vi "pco.camera_Simple_Example.vi"() -> ()   [LabVIEW 2019]
uses:
  pco.camera/Camera.lvclass
  <vilib>/picture/picture.llb/Draw 8-Bit Pixmap.vi
  <vilib>/picture/picture.llb/Draw True-Color Pixmap.vi
panel:
  out "colormap(U8)":u32[](array[numeric])
  out "Image(U16)":u16[][](graph)
  in  "Zoom [%]":i32(c297)=26
  out "Image":picture
  out "rawImage":u16[][](array[numeric])
  in  "data_format":T1(ring)=enum."Mono16"
  in  "Image Index":u32 max=9
  out "Recorded Images":u32
  in  "Quit":bool
  in  "roiY1":u64=2 min=2 max=2160 step=1
  in  "roiX1":u64=2 min=2 max=2560 step=1
  in  "roiY0":u64=1 min=1 max=2159 step=1
  in  "roiX0":u64=1 min=1 max=2559 step=1
  out "Image Height":u16
  out "Image Width":u16
  in  "dwImgCount":u32=10 caption="Required Number of Images" max=4023
  out "Error":errorcluster {"code" format="%x"}
  # "This example shows a simple recording of an image sequence and the image access afterwards.\nIt is a good starting point for writing own applications.\nBut it will not be fail save, i.e. doesnt react on errors, just handles them forward to the end\n\nUsage:\nSelect your required image count before you start the program.\nOnce started, the camera class will be initialized and images will be recorded automatically.\nWhen acquisition has finished you can address the images and set a certain roi \nTo finish the program click on quit application, this will force fan exit of the camera class"
  # "pco.labview"
  # "Camera Setup"
  # "Recording Control"
  # "Parameters for image readout"
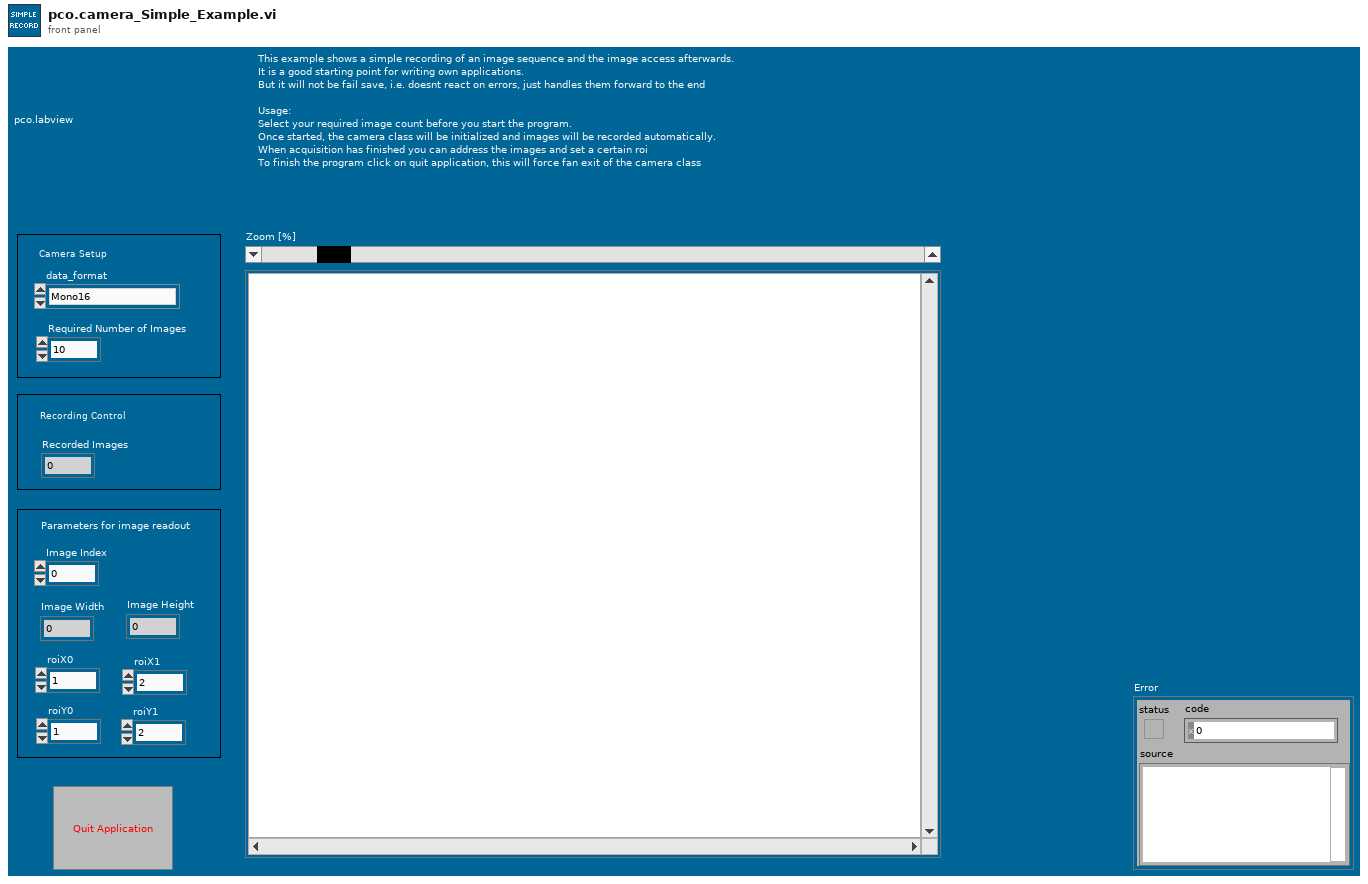
[diagram p1: front panel]
types:
  T1 = enum16{"Undefined", "Mono8", "Mono16", "BGRA8", "RGBA8", "BGRA16", "RGBA16", "CompressedMono8"}
  T2 = enum8{"Enabled", "Disabled", "Disabled and Grayed Out"}
  T3 = enum16{"sequence", "sequence non blocking", "ring buffer", "fifo", "sequence_dpcore", "sequence_non_blocking_dpcore", "ring_buffer_dpcore", "fifo_dpcore", "tif", "multitif", "pcoraw", "b16", "dicom", "multidicom"}
  T4 = typedef "Camera.lvclass/binning.ctl" = cluster{"vert":u16, "horz":u16}
  T5 = cluster{"exposure_time_s":dbl, "delay_time_s":dbl, "roi":cluster{"x0":u64, "y0":u64, "x1":u64, "y1":u64}, "timestamp_mode":u16, "pixelrate":u32, "trigger_mode":u16, "acquire_mode":u16, "metadata_mode":u16, "noisefilter_mode":u16, "binning":T4}
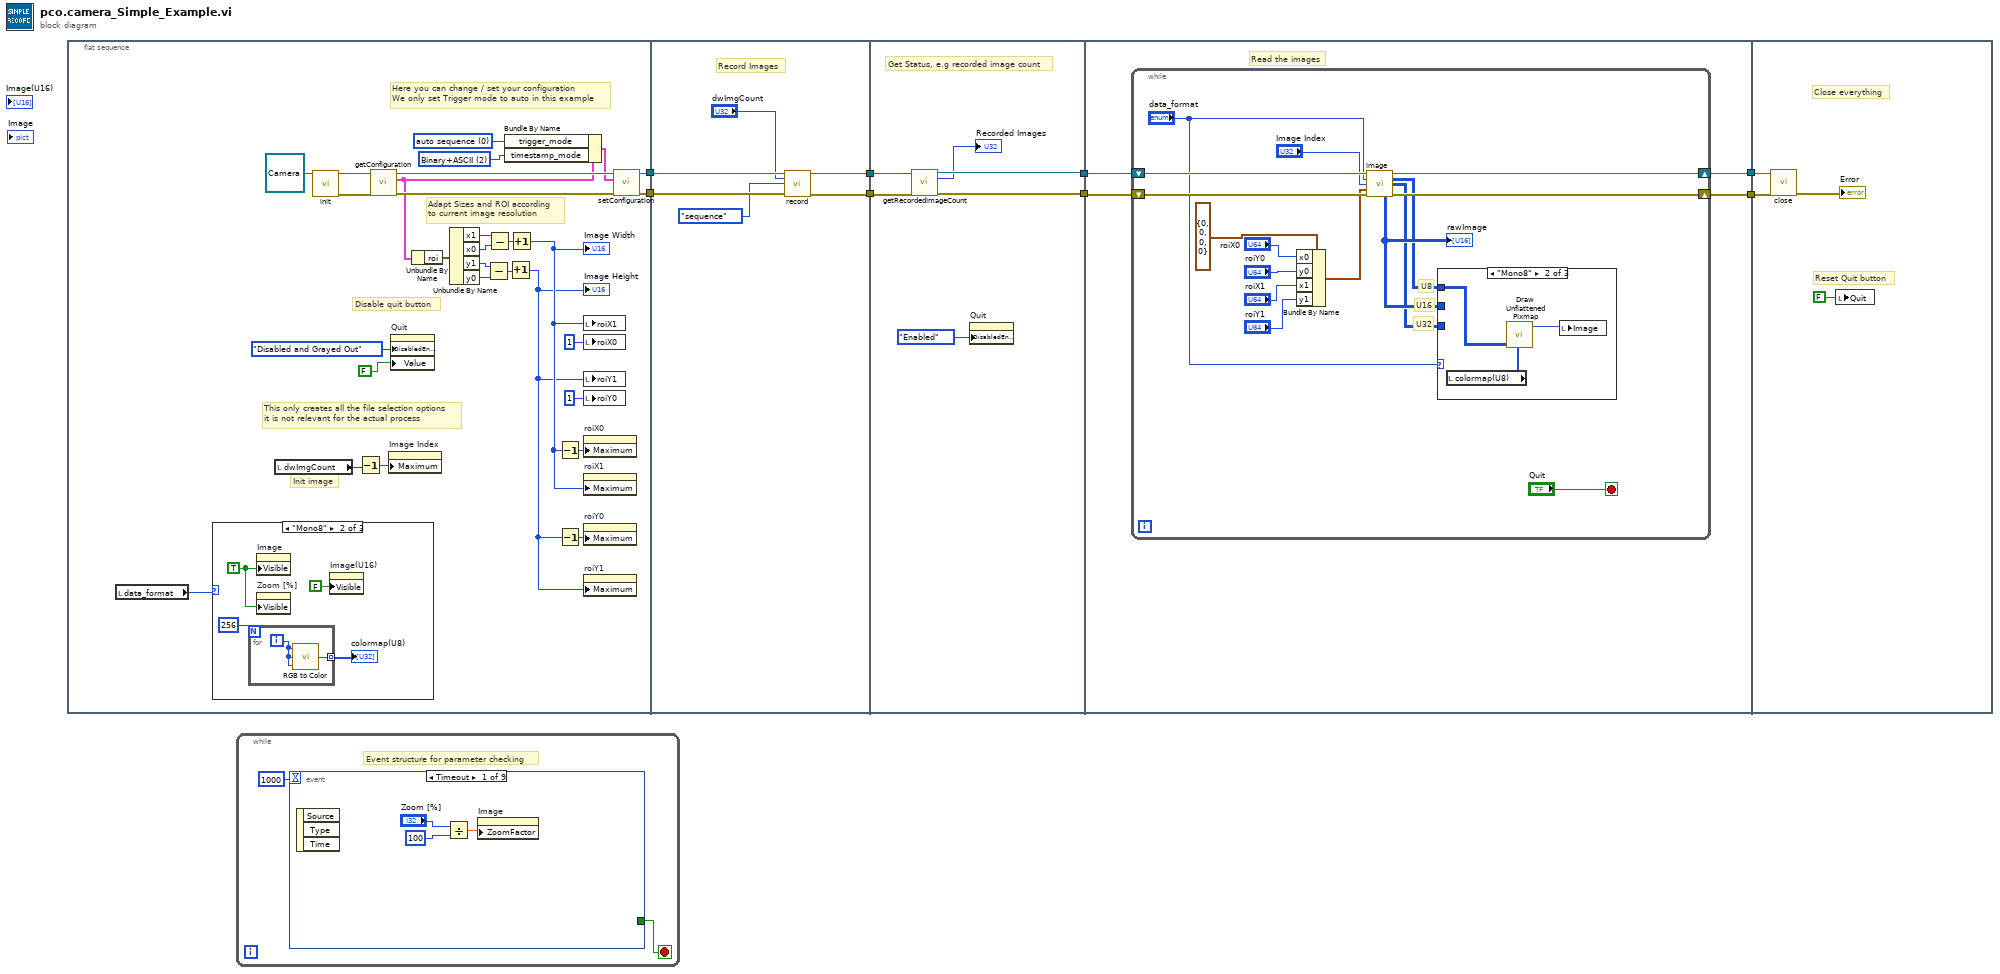
[diagram p0: block diagram]
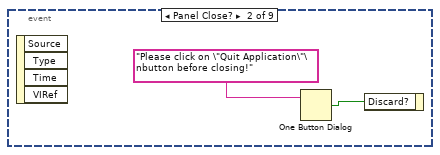
[diagram p2: hidden frame]
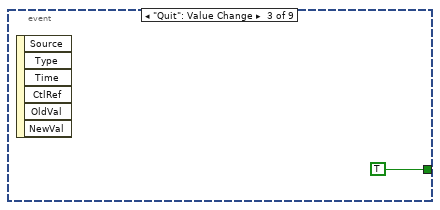
[diagram p3: hidden frame]
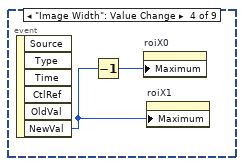
[diagram p4: hidden frame]
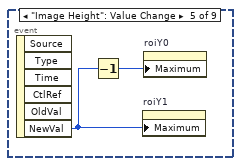
[diagram p5: hidden frame]
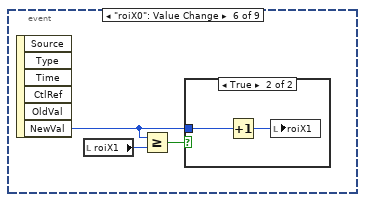
[diagram p6: hidden frame]
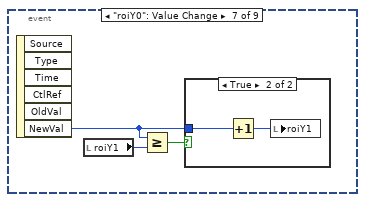
[diagram p8: hidden frame]
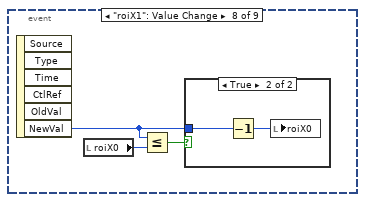
[diagram p10: hidden frame]
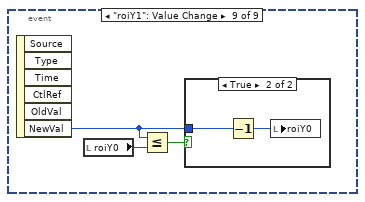
[diagram p12: hidden frame]
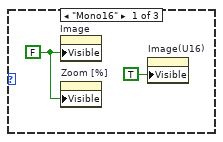
[diagram p14: hidden frame]
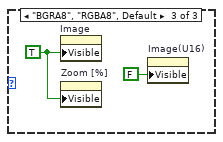
[diagram p15: hidden frame]
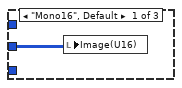
[diagram p16: hidden frame]
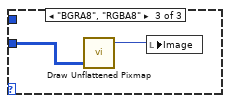
[diagram p17: hidden frame]
diagram:
  n1 = flat-sequence {
    tunnel: [w30] -> w8
    tunnel: [w29] -> w7
    tunnel: w8 -> [w53]
    tunnel: w7 -> [w52]
    tunnel: [w50] -> w6
    tunnel: [w49] -> w5
    tunnel: w6 -> [w59]
    tunnel: w5 -> [w58]
    tunnel: [w57] -> w4
    tunnel: [w56] -> w3
    tunnel: w4 -> [w62]
    tunnel: w3 -> [w63]
    tunnel: [w61] -> w2
    tunnel: [w60] -> w1
    tunnel: w2 -> [w87]
    tunnel: w1 -> [w86]
    frame #0 {
      w14 = u16 2 items=["OFF", "Binary", "Binary+ASCII", "ASCII"] ("TimestampMode")
      w34 = u16 0 items=["auto sequence"=0, "software trigger"=1, "external exposure start & software trigger"=2, "external exposure control"=3, "external synchronized"=4, "fast external exposure control"=5, "external CDS control"=6, "slow external exposure control"=7, "external synchronized HDSDI"=258] ("TriggerMode")
      # "Init image"
      # "This only creates all the file selection options\nit is not relevant for the actual process"
      # "Adapt Sizes and ROI according\nto current image resolution"
      # "Disable quit button"
      # "Here you can change / set your configuration\nWe only set Trigger mode to auto in this example"
      n2 = local read "data_format"() -> (w9:T1)
      n3 = case shown="\"Mono8\"" w9 {
        frame "Mono16" {
          w39 = FALSE ("Visible")
          n4 = property on="Image" class="Pict"("Visible"=w39) -> ()  [unwired: 2 in, 2 out]
          n5 = property on="Zoom [%]" class="Scroll (strict)"("Visible"=w39) -> ()  [unwired: 2 in, 2 out]
          n6 = property on="Image(U16)" class="IntGraph (strict)"("Visible"=TRUE) -> ()  [unwired: 2 in, 2 out]
        }
        frame "Mono8" {
          w42 = TRUE ("Visible")
          n7 = for {
            N: 256 -> [_]
            tunnel: [w44] -> w41 mode=indexing
            i -> [w45]
            n8 = call <vilib>:"RGB to Color.vi"("B"=w45, "G"=w45, "R"=w45) -> ("Color"=w44:u32)
          }
          "colormap(U8)" <- w41
          n9 = property on="Image" class="Pict"("Visible"=w42) -> ()  [unwired: 2 in, 2 out]
          n10 = property on="Zoom [%]" class="Scroll (strict)"("Visible"=w42) -> ()  [unwired: 2 in, 2 out]
          n11 = property on="Image(U16)" class="IntGraph (strict)"("Visible"=FALSE) -> ()  [unwired: 2 in, 2 out]
        }
        frame "BGRA8", "RGBA8", Default {
          w46 = TRUE ("Visible")
          n12 = property on="Image" class="Pict"("Visible"=w46) -> ()  [unwired: 2 in, 2 out]
          n13 = property on="Zoom [%]" class="Scroll (strict)"("Visible"=w46) -> ()  [unwired: 2 in, 2 out]
          n14 = property on="Image(U16)" class="IntGraph (strict)"("Visible"=FALSE) -> ()  [unwired: 2 in, 2 out]
        }
      }
      n15 = local read "dwImgCount"() -> (w10:u32)
      n16 = call-dynamic "init.vi"("Camera in"=refnum<class "Camera.lvclass"> refnum ("PCOCamera in")) -> ("Camera out"=w36:refnum<class "Camera.lvclass">, "error out"=w35:errorcluster)  [unwired: 8 in]
      n17 = Decrement(x=w10) -> (x-1=w11:u32)
      n18 = call-dynamic "getConfiguration.vi"("error in (no error)"=w35, "Camera in"=w36) -> ("error out"=w32:errorcluster, "configuration"=w24:T5, "Camera out"=w33:refnum<class "Camera.lvclass">)  [unwired: 7 in]
      n19 = property on="Image Index" class="DigNum (strict)"("Maximum"=w11) -> ()  [unwired: 2 in, 2 out]
      n20 = property on="Quit" class="Bool (strict)"("DisabledEnum"=T2."Disabled and Grayed Out" ("Disabled"), "Value"=FALSE ("Stop")) -> ()  [unwired: 2 in, 2 out]
      n21 = Unbundle By Name(w24) -> ("roi"=w23:cluster{"x0":u64, "y0":u64, "x1":u64, "y1":u64})
      n22 = Unbundle By Name(w23) -> ("x1"=w21:u64, "x0"=w22:u64, "y1"=w19:u64, "y0"=w20:u64)
      n23 = Subtract(x=w19, y=w20) -> (x-y=w17:u64)
      n24 = Subtract(x=w21, y=w22) -> (x-y=w18:u64)
      n25 = Bundle By Name(cluster=w24, "trigger_mode"=w34, "timestamp_mode"=w14) -> (w31:T5)
      n26 = Increment(x=w17) -> (x+1=w15:u64)
      "Image Height" <- w15
      n27 = Increment(x=w18) -> (x+1=w16:u64)
      "Image Width" <- w16
      n28 = Decrement(x=w16) -> (x-1=w26:u64)
      n29 = Decrement(x=w15) -> (x-1=w25:u64)
      n30 = local write "roiX1"(w16) -> ()
      n31 = local write "roiX0"(u16 1 ("roiY0")) -> ()
      n32 = local write "roiY1"(w15) -> ()
      n33 = local write "roiY0"(u16 1 ("roiY0")) -> ()
      n34 = property on="roiX0" class="DigNum (strict)"("Maximum"=w26) -> ()  [unwired: 2 in, 2 out]
      n35 = property on="roiX1" class="DigNum (strict)"("Maximum"=w16) -> ()  [unwired: 2 in, 2 out]
      n36 = property on="roiY0" class="DigNum (strict)"("Maximum"=w25) -> ()  [unwired: 2 in, 2 out]
      n37 = property on="roiY1" class="DigNum (strict)"("Maximum"=w15) -> ()  [unwired: 2 in, 2 out]
      n38 = call-dynamic "setConfiguration.vi"("error in (no error)"=w32, "configuration"=w31, "Camera in"=w33) -> ("error out"=w29:errorcluster, "Camera out"=w30:refnum<class "Camera.lvclass">)  [unwired: 7 in]
    }
    frame #1 {
      # "Record Images"
      n39 = call-dynamic "record.vi"("Camera in"=w53, "num_images"="dwImgCount", "record_mode"=T3."sequence", "error in (no error)"=w52) -> ("Camera out"=w50:refnum<class "Camera.lvclass">, "error out"=w49:errorcluster)  [unwired: 10 in]
    }
    frame #2 {
      # "Get Status, e.g recorded image count"
      n40 = call-dynamic "getRecordedImageCount.vi"("Camera in"=w59, "error in (no error)"=w58) -> ("Camera out"=w57:refnum<class "Camera.lvclass">, "recorded_image_count"=→"Recorded Images":u32, "error out"=w56:errorcluster)  [unwired: 11 in]
      n41 = property on="Quit" class="Bool (strict)"("DisabledEnum"=T2."Enabled" ("Disabled")) -> ()  [unwired: 2 in, 2 out]
    }
    frame #3 {
      # "Read the images"
      n42 = while {
        shift-right: [w77] -> w61
        shift-left: w62 -> [w79]
        shift-right: [w72] -> w60
        shift-left: w63 -> [w78]
        stop <- "Quit" stop-if-true
        # "U32"
        # "U16"
        # "U8"
        n43 = Bundle By Name(cluster=cluster{"x0":u64, "y0":u64, "x1":u64, "y1":u64} {"x0"=0, "y0"=0, "x1"=0, "y1"=0} ("roi"), "x0"="roiX0", "y0"="roiY0", "x1"="roiX1", "y1"="roiY1") -> (w71:cluster{"x0":u64, "y0":u64, "x1":u64, "y1":u64})
        n44 = call-dynamic "image.vi"("Camera in"=w79, "data_format"="data_format", "image_index"="Image Index", "roi"=w71, "error in (no error)"=w78) -> ("Camera out"=w77:refnum<class "Camera.lvclass">, "image (U8)"=w64:u8[][], "image (U32)"=w65:u32[][], "raw_image (U16)"=w66:u16[][], "error out"=w72:errorcluster)  [unwired: 3 in, 3 out]
        "rawImage" <- w66
        n45 = case shown="\"Mono8\"" "data_format" {
          tunnel: w65 -> [_ _ w85]
          tunnel: w64 -> [_ w82 _]
          tunnel: w66 -> [w80 _ _]
          frame "Mono16", Default {
            n46 = local write "Image(U16)"(w80) -> ()
          }
          frame "Mono8" {
            n47 = local read "colormap(U8)"() -> (w81:u32[])
            n48 = call-poly <vilib>:"Draw Unflattened Pixmap.vi"("data"=w82, "color table"=w81) -> ("new picture"=w83:picture)  [unwired: 7 in]
            n49 = local write "Image"(w83) -> ()
          }
          frame "BGRA8", "RGBA8" {
            n50 = call-poly <vilib>:"Draw Unflattened Pixmap.vi"("data (RGB format)"=w85) -> ("new picture"=w84:picture)  [unwired: 8 in]
            n51 = local write "Image"(w84) -> ()
          }
        }
      }
    }
    frame #4 {
      # "Reset Quit button"
      # "Close everything"
      n52 = call-dynamic "close.vi"("error in (no error)"=w86, "Camera in"=w87) -> ("error out"=→"Error":errorcluster)  [unwired: 9 in]
      n53 = local write "Quit"(FALSE ("Stop")) -> ()
    }
  }
  n54 = while {
    stop <- w90 stop-if-true
    # "Event structure for parameter checking"
    n55 = event shown="[0] Timeout" {
      selector: _ -> [_ _ _ _ _ _ _ _ _]
      dyn-events: _ -> [_ _ _ _ _ _ _ _ _]
      timeout: 1000 -> [_ _ _ _ _ _ _ _ _]
      tunnel: [_ _ TRUE _ _ _ _ _ _] -> w90
      event Timeout {
        n56 = event-data() -> ()  [unwired: 1 in, 3 out]
        n57 = Divide(x="Zoom [%]", y=100 ("Zoom [%]")) -> (x/y=w92:dbl)
        n58 = property on="Image" class="Pict"("ZoomFactor"=w92) -> ()  [unwired: 2 in, 2 out]
      }
      event Panel Close? {
        n59 = event-data() -> ()  [unwired: 1 in, 4 out]
        n60 = One Button Dialog(message="Please click on \"Quit Application\"\nbutton before closing!") -> (true=w95:bool)  [unwired: 1 in]
        n61 = event-data("Discard?"=w95) -> ()  [unwired: 1 in, 1 out]
      }
      event "Quit": Value Change {
        n62 = event-data() -> ()  [unwired: 1 in, 6 out]
      }
      event "Image Width": Value Change {
        n63 = event-data() -> ("NewVal"=w98:u16)  [unwired: 1 in, 5 out]
        n64 = Decrement(x=w98) -> (x-1=w99:u16)
        n65 = property on="roiX0" class="DigNum (strict)"("Maximum"=w99) -> ()  [unwired: 2 in, 2 out]
        n66 = property on="roiX1" class="DigNum (strict)"("Maximum"=w98) -> ()  [unwired: 2 in, 2 out]
      }
      event "Image Height": Value Change {
        n67 = event-data() -> ("NewVal"=w100:u16)  [unwired: 1 in, 5 out]
        n68 = Decrement(x=w100) -> (x-1=w101:u16)
        n69 = property on="roiY1" class="DigNum (strict)"("Maximum"=w100) -> ()  [unwired: 2 in, 2 out]
        n70 = property on="roiY0" class="DigNum (strict)"("Maximum"=w101) -> ()  [unwired: 2 in, 2 out]
      }
      event "roiX0": Value Change {
        n71 = event-data() -> ("NewVal"=w102:u64)  [unwired: 1 in, 5 out]
        n72 = local read "roiX1"() -> (w104:u64)
        n73 = Greater Or Equal?(x=w102, y=w104) -> (x >= y?=w103:bool)
        n74 = case shown="True" w103 {
          tunnel: w102 -> [_ w106]
          frame False {
          }
          frame True {
            n75 = Increment(x=w106) -> (x+1=w105:u64)
            n76 = local write "roiX1"(w105) -> ()
          }
        }
      }
      event "roiY0": Value Change {
        n77 = event-data() -> ("NewVal"=w107:u64)  [unwired: 1 in, 5 out]
        n78 = local read "roiY1"() -> (w109:u64)
        n79 = Greater Or Equal?(x=w107, y=w109) -> (x >= y?=w108:bool)
        n80 = case shown="True" w108 {
          tunnel: w107 -> [_ w111]
          frame False {
          }
          frame True {
            n81 = Increment(x=w111) -> (x+1=w110:u64)
            n82 = local write "roiY1"(w110) -> ()
          }
        }
      }
      event "roiX1": Value Change {
        n83 = event-data() -> ("NewVal"=w112:u64)  [unwired: 1 in, 5 out]
        n84 = local read "roiX0"() -> (w114:u64)
        n85 = Less Or Equal?(x=w112, y=w114) -> (x <= y?=w113:bool)
        n86 = case shown="True" w113 {
          tunnel: w112 -> [_ w116]
          frame False {
          }
          frame True {
            n87 = Decrement(x=w116) -> (x-1=w115:u64)
            n88 = local write "roiX0"(w115) -> ()
          }
        }
      }
      event "roiY1": Value Change {
        n89 = event-data() -> ("NewVal"=w117:u64)  [unwired: 1 in, 5 out]
        n90 = local read "roiY0"() -> (w119:u64)
        n91 = Less Or Equal?(x=w117, y=w119) -> (x <= y?=w118:bool)
        n92 = case shown="True" w118 {
          tunnel: w117 -> [_ w121]
          frame False {
          }
          frame True {
            n93 = Decrement(x=w121) -> (x-1=w120:u64)
            n94 = local write "roiY0"(w120) -> ()
          }
        }
      }
    }
  }
